vi "close_listener.vi"(0 "zmq_mlt in":refnum<class "zmq_multipart_lib.lvclass">, 11 "error in (no error)":errorcluster) -> (4 "zmq_mlt out":refnum<class "zmq_multipart_lib.lvclass">, 15 "error out":errorcluster)   [LabVIEW 2019, in "zmq_multipart_lib.lvlib" / "zmq_multipart_lib.lvclass"]
uses:
  zmq_multipart_lib.lvclass
  zmq_multipart_lib.lvclass/zmq_multipart_lib.ctl
  <vilib>/addons/zeromq/zmq_socket.lvclass
  <vilib>/addons/zeromq/zeromq.lvlib
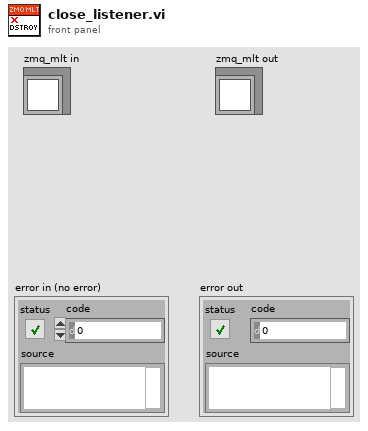
[diagram p1: front panel]
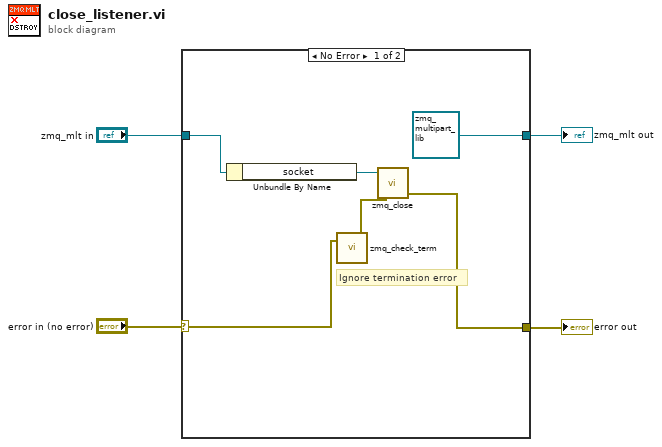
[diagram p0: block diagram]
diagram:
  n1 = case shown="No Error" "error in (no error)" {
    selector: "error in (no error)" -> [w7 w12]
    tunnel: [w6 w12] -> w4
    tunnel: "zmq_mlt in" -> [w10 w11]
    tunnel: [refnum<class "zmq_multipart_lib.lvclass"> refnum ("zmq_mlt in") w11] -> w2
    frame No Error {
      # "Ignore termination error"
      n2 = Unbundle By Name(w10) -> ("socket"=w8:refnum<class "zmq_socket.lvclass">)
      n3 = call <vilib>:"zmq_check_term.vi"("error in"=w7) -> ("error out"=w9:errorcluster)  [unwired: 1 in, 1 out]
      n4 = call <vilib>:"zmq_close.vi"("error in"=w9, "socket"=w8) -> ("error out"=w6:errorcluster)  [unwired: 3 in]
    }
    frame Error {
    }
  }
  "error out" <- w4
  "zmq_mlt out" <- w2
